vi "DB_ChooseModule.vi"(8 "error in":errorcluster, 11 "路径 in":path) -> (0 "error out":errorcluster, 1 "Config":T1, 2 "型号 2":string(combo), 3 "OK?":bool)   [LabVIEW 2013, in "Settings-Style.lvlib"]
uses:
  Settings-Style.lvlib
  1_Ctl/DB_UUT.ctl
  1_ctl/Ctl-Color.ctl
panel:
  in  "Cancel Button":bool
  in  "OK Button":bool
  in  "型号":string(combo)
  # "请选择待测试产品型号！"
  # "Style Settings"
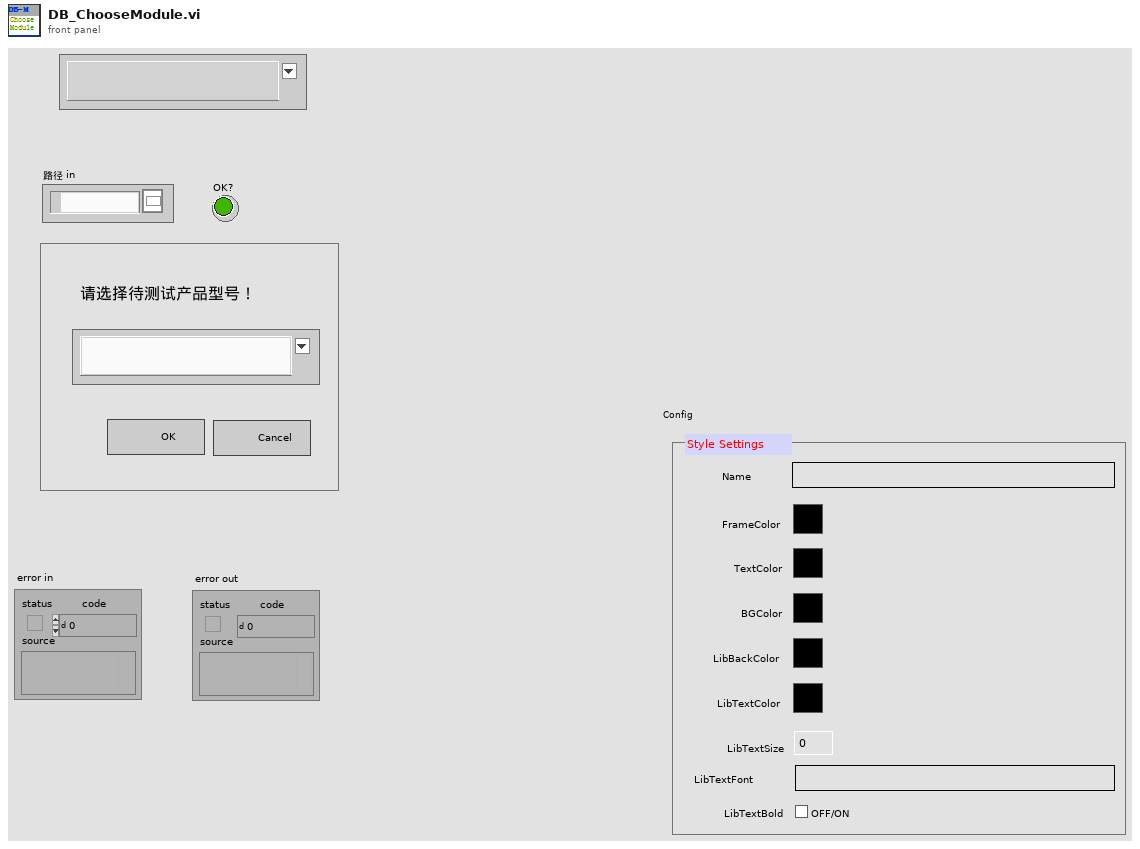
[diagram p1: front panel]
types:
  T1 = typedef "Settings-Style.lvlib/DB_UUT.ctl" = cluster{"Name":string, "FrameColor":T2, "TextColor":T2, "BGColor":T2, "LibBackColor":T2, "LibTextColor":T2, "LibTextSize":u32, "LibTextFont":string, "LibTextBold":bool}
  T2 = typedef "Ctl-Color.ctl" = u32
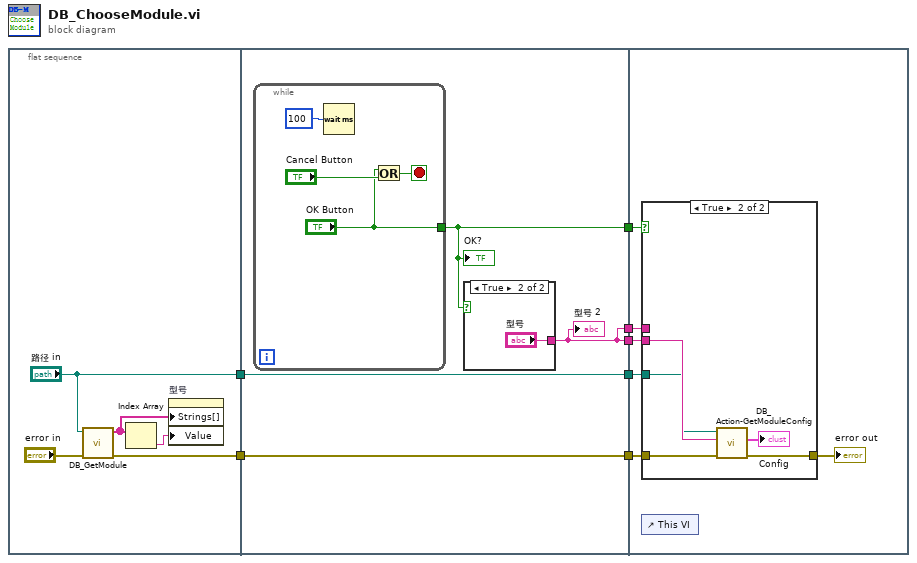
[diagram p0: block diagram]
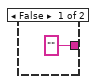
[diagram p2: hidden frame]
diagram:
  n1 = flat-sequence {
    tunnel: ["路径 in"] -> w4
    tunnel: [w10] -> w3
    tunnel: [w14] -> w7
    tunnel: w4 -> [w16]
    tunnel: [w16] -> w6
    tunnel: w3 -> [w15]
    tunnel: [w15] -> w5
    tunnel: [w14] -> w2
    tunnel: [w13] -> w1
    tunnel: w7 -> [w28]
    tunnel: w6 -> [w27]
    tunnel: w5 -> [w26]
    tunnel: w2 -> [w24]
    tunnel: w1 -> [w23]
    frame #0 {
      n2 = call "DB_GetModule.vi"("error in (no error)"="error in", 11:"路径 in") -> ("error out"=w10:errorcluster, "Data"=w9:string[])  [unwired: 8 in]
      n3 = Index Array(array=w9) -> (element=w8:string)  [unwired: 1 in]
      n4 = property on="型号" class="CmbBox"("Strings[]"=w9, "Value"=w8) -> ()  [unwired: 2 in, 2 out]
    }
    frame #1 {
      n5 = while {
        tunnel: ["OK Button"] -> w13
        stop <- w21 stop-if-true
        n6 = Wait (ms)(milliseconds to wait=u32 100) -> ()  [unwired: 1 out]
        n7 = Or(x="OK Button", y="Cancel Button") -> (x .or. y?=w21:bool)
      }
      "OK?" <- w13
      n8 = case shown="True" w13 {
        tunnel: ["" ("型号") "型号"] -> w14
        frame False {
        }
        frame True {
        }
      }
      "型号 2" <- w14
    }
    frame #2 {
      n9 = case shown="True" w23 {
        tunnel: w28 -> [_ w34]
        tunnel: w27 -> [_ w33]
        tunnel: w26 -> [w29 w32]
        tunnel: [w29 w30] -> w25
        tunnel: w24 -> [_ _]
        frame False {
        }
        frame True {
          n10 = call "DB_Action-GetModuleConfig.vi"("error in"=w32, 10:w34, "Name"=w33) -> ("error out"=w30:errorcluster, "Config"=→"Config":T1)  [unwired: 6 in, 1 out]
        }
      }
      "error out" <- w25
      n11 = control-ref of="This VI"() -> ()  [unwired: 1 out]
    }
  }
